vi "Fetch Min Max Waveform.vi"(8 "error in (no error)":errorcluster {"code" format="%.0x"}, 10 "Channel Name (\"Channel 1\")":string(combo)="CHAN1", 11 "VISA Resource Name":refnum<visa-resource-name>) -> (0 "error out":errorcluster {"code" format="%.0x"}, 1 "x increment":dbl caption="x Increment" format="%^.2e", 2 "initial x":dbl caption="Initial x" format="%^.2e", 3 "VISA Resource Name Out":refnum<visa-resource-name>, 4 "Max waveform array":dbl[](array[numeric]) caption="Max Waveform Array" format="%.2f", 5 "actual points":u32 caption="Actual Points", 6 "Min waveform array":dbl[](array[numeric]) caption="Min Waveform Array" format="%.2f")   [LabVIEW 2011, in "Agilent 546XX Series.lvlib"]
doc: "This VI returns the minimum and maximum waveforms that the oscilloscope acquires for the channel you specify. The waveforms are from an acquisition that you previously initiated. Use this VI to fetch waveforms when you set the acquisition type to Peak Detect.\n\nUse the ag546xx Initiate Acquisition VI to start an acquisition on the channels that you enable with the ag546xx Configure Channel VI. The oscilloscope acquires the min/max waveforms for the enabled channels concurrently. You use the ag546xx Acquisition Status VI to determine when the acquisition is complete. You must call this VI separately for each enabled channel to obtain the min/max waveforms.\n\nYou can call the ag546xx Read Min Max Waveform VI instead of the ag546xx Initiate Acquisition VI. The ag546xx Read Min Max Waveform VI starts an acquisition on all enabled channels, waits for the acquisition to complete, and returns the min/max waveforms for the channel you specify. You call this VI to obtain the min/max waveforms for each of the remaining channels.\n\nNotes:\n\n(1) After this VI executes, each element in the Min Waveform Array and Max Waveform Array is either a voltage or a value indicating that the oscilloscope could not sample a voltage.\n\n(2) This VI does not check the instrument status. Typically, you call this VI only in a sequence of calls to other low-level driver VIs. The sequence performs one operation. You use the low-level VIs to optimize one or more aspects of interaction with the instrument. If you want to check the instrument status, call the ag546xx Error-Query VI at the conclusion of the sequence."
uses:
  Agilent 546XX Series.lvlib
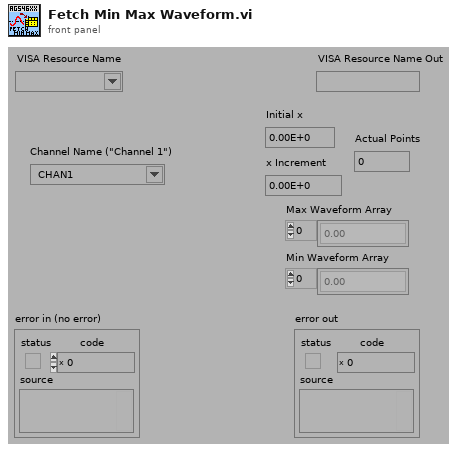
[diagram p1: front panel]
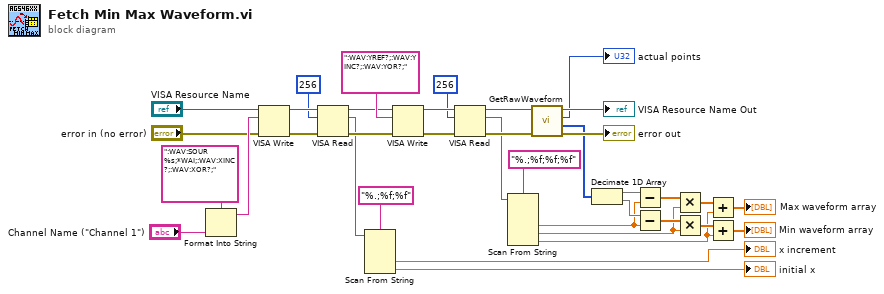
[diagram p0: block diagram]
diagram:
  n1 = Format Into String(format string=":WAV:SOUR %s;*WAI;:WAV:XINC?;:WAV:XOR?;", "Channel Name (\"Channel 1\")") -> (resulting string=w36:string)  [unwired: 2 in, 1 out]
  n2 = VISA Write(VISA resource name="VISA Resource Name", write buffer=w36, error in (no error)="error in (no error)") -> (VISA resource name out=w9:refnum<visa-resource-name>, error out=w7:errorcluster)  [unwired: 1 out]
  n3 = VISA Read(VISA resource name=w9, byte count=u32 256, error in (no error)=w7) -> (VISA resource name out=w5:refnum<visa-resource-name>, read buffer=w3:string, error out=w6:errorcluster)  [unwired: 1 out]
  n4 = Scan From String(format string="%.;%f;%f", input string=w3) -> (output 1=→"x increment":dbl, output 2=→"initial x":dbl)  [unwired: 4 in, 3 out]
  n5 = VISA Write(VISA resource name=w5, write buffer=":WAV:YREF?;:WAV:YINC?;:WAV:YOR?;", error in (no error)=w6) -> (VISA resource name out=w35:refnum<visa-resource-name>, error out=w34:errorcluster)  [unwired: 1 out]
  n6 = VISA Read(VISA resource name=w35, byte count=u32 256, error in (no error)=w34) -> (VISA resource name out=w33:refnum<visa-resource-name>, read buffer=w27:string, error out=w32:errorcluster)  [unwired: 1 out]
  n7 = Scan From String(format string="%.;%f;%f;%f", input string=w27) -> (output 1=w15:dbl, output 2=w17:dbl, output 3=w16:dbl)  [unwired: 5 in, 3 out]
  n8 = call "GetRawWaveform.vi"("error in"=w32, "VISA Resource Name"=w33) -> ("error out"=→"error out":errorcluster, "Waveform Array"=w22:u32[], "Number of Points"=→"actual points":u32, "VISA Resource Name Out"=→"VISA Resource Name Out":refnum<visa-resource-name>)  [unwired: 5 in, 1 out]
  n9 = Decimate 1D Array(w22) -> (w18:u32[], w21:u32[])
  n10 = Subtract(x=w18, y=w15) -> (x-y=w19:dbl[])
  n11 = Subtract(x=w21, y=w15) -> (x-y=w25:dbl[])
  n12 = Multiply(x=w19, y=w17) -> (x*y=w20:dbl[])
  n13 = Multiply(x=w25, y=w17) -> (x*y=w24:dbl[])
  n14 = Add(x=w20, y=w16) -> (x+y=→"Max waveform array":dbl[])
  n15 = Add(x=w24, y=w16) -> (x+y=→"Min waveform array":dbl[])
